vi "Give old config to New config.vi"() -> ()   [LabVIEW 2022 SP3]
uses:
  Controls/SeCrTs-Config.ctl
panel:
  in  "Config 2":T1={"AO config"=[], "AI config"=[], "DI config"=[], "DO config"=[], "TC config"=[{"Channel_Name"="", "Channel_Number"="", "Pre_Scale_min"=0.0, "Pre_Scale_max"=0.0, "units"=4, " type"=7}], "ACC config"=[], "SG config"=[], "Strain Gauge Settings"={"poisson ratio"=0.3, "nominal gage resistance"=120.0, "gage factor"=2.08}, "Bridge Settings"={"voltage excitation value"=3.3, "voltage excitation source"=10200, "initial bridge voltage"=0.0, "lead wire resistance"=1.7, "strain configuration"=10271}, "Sample Rate"={"AI Sample Rate"=[], "AO Sample Rate"=[], "DI Sample Rate"=[], "TC Sample Rate"=[], "DO Sample Rate"=[], "SG Sample Rate"=[], "ACC Sample Rate"=[]}} {"Bridge Settings"."strain configuration" items=["Full Bridge I"=10183, "Full Bridge II"=10184, "Full Bridge III"=10185, "Half Bridge I"=10188, "Half Bridge II"=10189, "Quarter Bridge I"=10271, "Quarter Bridge II"=10272]; "Bridge Settings"."voltage excitation source" items=["Internal"=10200, "External"=10167, "None"=10230]; "ACC config"."Terminal configuration" items=["default"=-1, "RSE"=10083, "NRSE"=10078, "Differential"=10106, "Pseudodifferential"=12529]; "ACC config"."Sensitivity units" items=["mVolts/g"=12509, "Volts/g"=12510]; "TC config"."type" items=["J"=10072, "K"=10073, "N"=10077, "R"=10082, "S"=10085, "T"=10086, "B"=10047, "E"=10055]; "TC config"."units" items=["Deg C", "Deg F", "Kelvins", "Deg R", "From Custom Scale"]}
  out "output cluster":T1={"AO config"=[], "AI config"=[], "DI config"=[], "DO config"=[], "TC config"=[], "ACC config"=[], "SG config"=[], "Strain Gauge Settings"={"poisson ratio"=0.3, "nominal gage resistance"=120.0, "gage factor"=2.08}, "Bridge Settings"={"voltage excitation value"=3.3, "voltage excitation source"=10200, "initial bridge voltage"=0.0, "lead wire resistance"=1.7, "strain configuration"=10271}, "Sample Rate"={"AI Sample Rate"=[], "AO Sample Rate"=[], "DI Sample Rate"=[], "TC Sample Rate"=[], "DO Sample Rate"=[], "SG Sample Rate"=[], "ACC Sample Rate"=[]}} {"Bridge Settings"."strain configuration" items=["Full Bridge I"=10183, "Full Bridge II"=10184, "Full Bridge III"=10185, "Half Bridge I"=10188, "Half Bridge II"=10189, "Quarter Bridge I"=10271, "Quarter Bridge II"=10272]; "Bridge Settings"."voltage excitation source" items=["Internal"=10200, "External"=10167, "None"=10230]; "ACC config"."Terminal configuration" items=["default"=-1, "RSE"=10083, "NRSE"=10078, "Differential"=10106, "Pseudodifferential"=12529]; "ACC config"."Sensitivity units" items=["mVolts/g"=12509, "Volts/g"=12510]; "TC config"."type" items=["J"=10072, "K"=10073, "N"=10077, "R"=10082, "S"=10085, "T"=10086, "B"=10047, "E"=10055]; "TC config"."units" items=["Deg C", "Deg F", "Kelvins", "Deg R", "From Custom Scale"]}
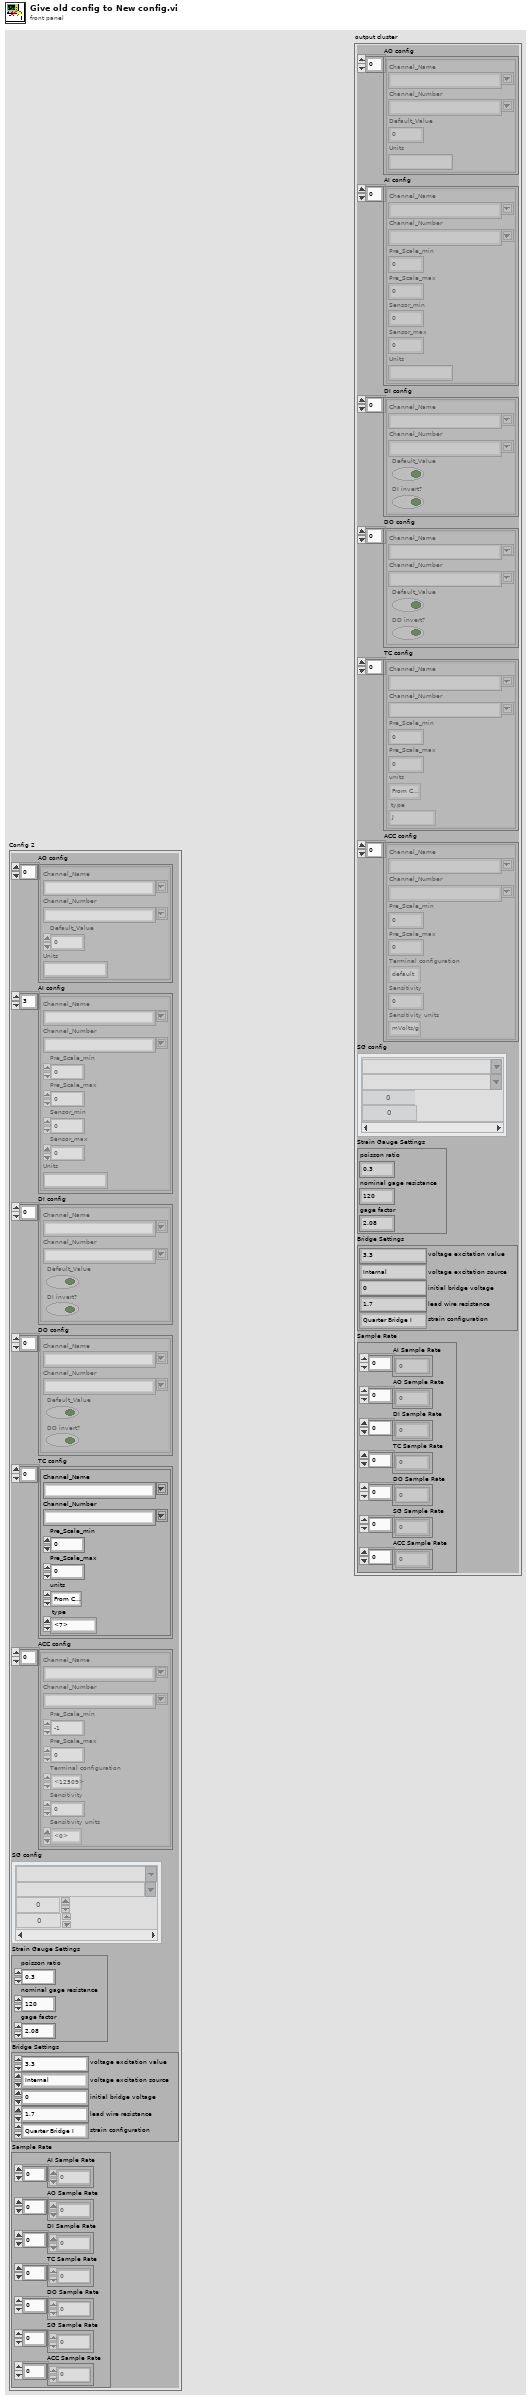
[diagram p1: front panel]
types:
  T1 = typedef "SeCrTs-Config.ctl" = cluster{"AO config":cluster{"Channel_Name":string, "Channel_Number":string, "Default_Value":dbl, "Units":string}[], "AI config":cluster{"Channel_Name":string, "Channel_Number":string, "Pre_Scale_min":dbl, "Pre_Scale_max":dbl, "Sensor_min":dbl, "Sensor_max":dbl, "Units":string}[], "DI config":cluster{"Channel_Name":string, "Channel_Number":string, "Default_Value":bool, "DI invert?":bool}[], "DO config":cluster{"Channel_Name":string, "Channel_Number":string, "Default_Value":bool, "DO invert?":bool}[], "TC config":cluster{"Channel_Name":string, "Channel_Number":string, "Pre_Scale_min":dbl, "Pre_Scale_max":dbl, "units":i32, " type":i32}[], "ACC config":cluster{"Channel_Name":string, "Channel_Number":string, "Pre_Scale_min":dbl, "Pre_Scale_max":dbl, "Terminal configuration":i32, "Sensitivity":dbl, "Sensitivity units":i32}[], "SG config":cluster{"Channel_Name":string, "Channel_Number":string, "Pre_Scale_min":dbl, "Pre_Scale_max":dbl}[], "Strain Gauge Settings":cluster{"poisson ratio":dbl, "nominal gage resistance":dbl, "gage factor":dbl}, "Bridge Settings":cluster{"voltage excitation value":dbl, "voltage excitation source":i32, "initial bridge voltage":dbl, "lead wire resistance":dbl, "strain configuration":i32}, "Sample Rate":cluster{"AI Sample Rate":dbl[], "AO Sample Rate":dbl[], "DI Sample Rate":dbl[], "TC Sample Rate":dbl[], "DO Sample Rate":dbl[], "SG Sample Rate":dbl[], "ACC Sample Rate":dbl[]}}
  T2 = cluster{cluster{"AI":cluster{"AI signal Lists":string, "AI Channel List":string, "Prescale Min":dbl, "Prescale Max":dbl, "Prescale Unit":string, "Sensor Min":dbl, "Sensor Max":dbl, "Sensor Unit":string}[], "AI Sample rate":u32[], "AI Device list ":string[]}, cluster{"AO":cluster{"AO signal List":string, "AO Channel List":string, "AO Default Value":dbl}[], "AO Sample rate ":u32[], "AO Device list":string[]}, cluster{"DI":cluster{"DI Signal List":string, "DI Channel list":string, "Default":bool, "Inverted":bool}[], "DI Sample rate":u32[], "DI Device list  ":string[]}, cluster{"DO":cluster{"DO Signal List":string, "DO Channel List":string, "DO Default":bool, "DO Inverted":bool}[], "DO Sample rate":u32[], "DO Device list ":string[]}, cluster{"CI":cluster{"CI Signal list":string, "CI Channel List":string, "Initial Count":u32, "Count Direction":i32, "Edge":i32}[], "CI Sample rate":u32[], "CI Device list ":string[]}, cluster{"TC":cluster{"TC signal Lists":string, "TC Channel Lists":string, "TC type":i32, "Max.Value":dbl, "Min.Value":dbl, "Units":i32}[], "TC Sample rate":u32[], "TC Device list":string[]}, cluster{"Accelerometer":cluster{"name to assign":string, "physical channels":tag, "minimum value":dbl, "maximum value":dbl, "sensitivity":dbl, "sensitivity units":i32, "units":i32}[], "Acc Sampling Rate":string}}
  T3 = cluster{"AI":cluster{"AI signal Lists":string, "AI Channel List":string, "Prescale Min":dbl, "Prescale Max":dbl, "Prescale Unit":string, "Sensor Min":dbl, "Sensor Max":dbl, "Sensor Unit":string}[], "AI Sample rate":u32[], "AI Device list ":string[]}
  T4 = cluster{"AO":cluster{"AO signal List":string, "AO Channel List":string, "AO Default Value":dbl}[], "AO Sample rate ":u32[], "AO Device list":string[]}
  T5 = cluster{"DI":cluster{"DI Signal List":string, "DI Channel list":string, "Default":bool, "Inverted":bool}[], "DI Sample rate":u32[], "DI Device list  ":string[]}
  T6 = cluster{"DO":cluster{"DO Signal List":string, "DO Channel List":string, "DO Default":bool, "DO Inverted":bool}[], "DO Sample rate":u32[], "DO Device list ":string[]}
  T7 = cluster{"TC":cluster{"TC signal Lists":string, "TC Channel Lists":string, "TC type":i32, "Max.Value":dbl, "Min.Value":dbl, "Units":i32}[], "TC Sample rate":u32[], "TC Device list":string[]}
  T8 = cluster{"Accelerometer":cluster{"name to assign":string, "physical channels":tag, "minimum value":dbl, "maximum value":dbl, "sensitivity":dbl, "sensitivity units":i32, "units":i32}[], "Acc Sampling Rate":string}
  T9 = cluster{"name to assign":string, "physical channels":tag, "minimum value":dbl, "maximum value":dbl, "sensitivity":dbl, "sensitivity units":i32, "units":i32}[]
  T10 = cluster{"AO signal List":string, "AO Channel List":string, "AO Default Value":dbl}[]
  T11 = cluster{"DO Signal List":string, "DO Channel List":string, "DO Default":bool, "DO Inverted":bool}[]
  T12 = cluster{"TC signal Lists":string, "TC Channel Lists":string, "TC type":i32, "Max.Value":dbl, "Min.Value":dbl, "Units":i32}[]
  T13 = cluster{"AI signal Lists":string, "AI Channel List":string, "Prescale Min":dbl, "Prescale Max":dbl, "Prescale Unit":string, "Sensor Min":dbl, "Sensor Max":dbl, "Sensor Unit":string}[]
  T14 = cluster{"DI Signal List":string, "DI Channel list":string, "Default":bool, "Inverted":bool}[]
  T15 = cluster{"Channel_Name":string, "Channel_Number":string, "Pre_Scale_min":dbl, "Pre_Scale_max":dbl, "units":i32, " type":i32}
  T16 = cluster{"Channel_Name":string, "Channel_Number":string, "Pre_Scale_min":dbl, "Pre_Scale_max":dbl, "Sensor_min":dbl, "Sensor_max":dbl, "Units":string}
  T17 = cluster{"Channel_Name":string, "Channel_Number":string, "Default_Value":dbl, "Units":string}
  T18 = cluster{"Channel_Name":string, "Channel_Number":string, "Default_Value":bool, "DI invert?":bool}
  T19 = cluster{"Channel_Name":string, "Channel_Number":string, "Pre_Scale_min":dbl, "Pre_Scale_max":dbl, "Terminal configuration":i32, "Sensitivity":dbl, "Sensitivity units":i32}
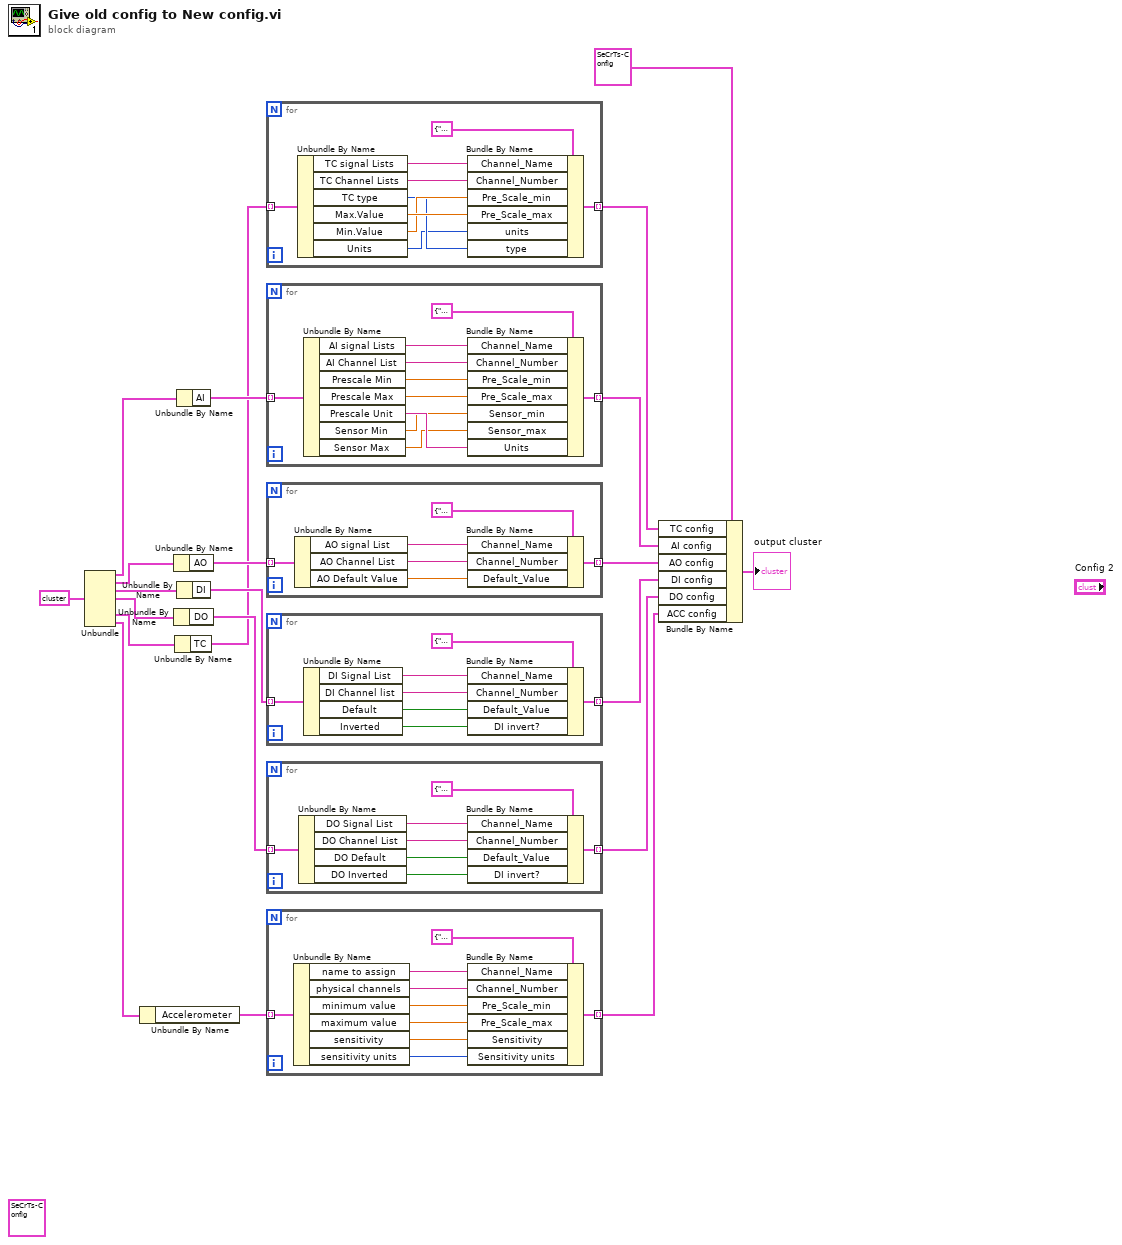
[diagram p0: block diagram]
diagram:
  (unwired) T1 {"AO config"=[{"Channel_Name"="TCV_1018", "Channel_Number"="PXI1Slot6/ao0", "Default_Value"=0.0, "Units"="Volt"}], "AI config"=[{"Channel_Name"="F_PT_1019", "Channel_Number"="PXI1Slot10/ai1", "Pre_Scale_min"=0.004, "Pre_Scale_max"=0.02, "Sensor_min"=0.0, "Sensor_max"=40.0, "Units"="bar"}, {"Channel_Name"="F_RTD_1013", "Channel_Number"="PXI1Slot10/ai2", "Pre_Scale_min"=0.004, "Pre_Scale_max"=0.02, "Sensor_min"=73.15, "Sensor_max"=373.15, "Units"="K"}, {"Channel_Name"="F_PT_1013a", "Channel_Number"="PXI1Slot10/ai3", "Pre_Scale_min"=0.004, "Pre_Scale_max"=0.02, "Sensor_min"=0.0, "Sensor_max"=200.0, "Units"="bar"}, {"Channel_Name"="F_PT_1013b", "Channel_Number"="PXI1Slot10/ai4", "Pre_Scale_min"=0.004, "Pre_Scale_max"=0.02, "Sensor_min"=0.0, "Sensor_max"=200.0, "Units"="bar"}, {"Channel_Name"="F_PT_1011a", "Channel_Number"="PXI1Slot10/ai5", "Pre_Scale_min"=0.004, "Pre_Scale_max"=0.02, "Sensor_min"=0.0, "Sensor_max"=40.0, "Units"="bar"}, {"Channel_Name"="F_PT_1011b", "Channel_Number"="PXI1Slot10/ai6", "Pre_Scale_min"=0.004, "Pre_Scale_max"=0.02, "Sensor_min"=0.0, "Sensor_max"=40.0, "Units"="bar"}, {"Channel_Name"="F_SC_RTD", "Channel_Number"="PXI1Slot10/ai7", "Pre_Scale_min"=0.004, "Pre_Scale_max"=0.02, "Sensor_min"=73.15, "Sensor_max"=373.15, "Units"="K"}, {"Channel_Name"="W_RTD_1177", "Channel_Number"="PXI1Slot10/ai8", "Pre_Scale_min"=0.004, "Pre_Scale_max"=0.02, "Sensor_min"=73.15, "Sensor_max"=773.15, "Units"="K"}, {"Channel_Name"="N_PT_1090", "Channel_Number"="PXI1Slot10/ai10", "Pre_Scale_min"=0.004, "Pre_Scale_max"=0.02, "Sensor_min"=0.0, "Sensor_max"=40.0, "Units"="bar"}, {"Channel_Name"="TCV_1018(FB)", "Channel_Number"="PXI1Slot10/ai11", "Pre_Scale_min"=0.004, "Pre_Scale_max"=0.02, "Sensor_min"=0.0, "Sensor_max"=100.0, "Units"="Percentage"}, {"Channel_Name"="F_FM-1010", "Channel_Number"="PXI1Slot10/ai12", "Pre_Scale_min"=0.004, "Pre_Scale_max"=0.02, "Sensor_min"=0.0, "Sensor_max"=10.0, "Units"="kg/s"}, {"Channel_Name"="F_PT_SC", "Channel_Number"="PXI1Slot10/ai13", "Pre_Scale_min"=0.004, "Pre_Scale_max"=0.02, "Sensor_min"=0.0, "Sensor_max"=40.0, "Units"="bar"}, {"Channel_Name"="PT 1000 - 2", "Channel_Number"="PXI1Slot10/ai14", "Pre_Scale_min"=0.004, "Pre_Scale_max"=0.02, "Sensor_min"=253.15, "Sensor_max"=453.15, "Units"="K"}, {"Channel_Name"="PT 1000 ", "Channel_Number"="PXI1Slot10/ai17", "Pre_Scale_min"=0.004, "Pre_Scale_max"=0.02, "Sensor_min"=253.15, "Sensor_max"=453.15, "Units"="K"}, {"Channel_Name"="N_PT_1101", "Channel_Number"="cRIOMod3/ai0", "Pre_Scale_min"=0.0, "Pre_Scale_max"=10.0, "Sensor_min"=0.0, "Sensor_max"=40.0, "Units"="bar"}, {"Channel_Name"="N_PT_1210", "Channel_Number"="cRIOMod3/ai1", "Pre_Scale_min"=0.0, "Pre_Scale_max"=10.0, "Sensor_min"=0.0, "Sensor_max"=100.0, "Units"="bar"}, {"Channel_Name"="W_PT_1212", "Channel_Number"="cRIOMod3/ai2", "Pre_Scale_min"=0.0, "Pre_Scale_max"=10.0, "Sensor_min"=0.0, "Sensor_max"=100.0, "Units"="bar"}, {"Channel_Name"="F_RTD_1212", "Channel_Number"="cRIOMod3/ai3", "Pre_Scale_min"=0.0, "Pre_Scale_max"=10.0, "Sensor_min"=73.15, "Sensor_max"=373.15, "Units"="K"}, {"Channel_Name"="Tank6", "Channel_Number"="cRIOMod3/ai4", "Pre_Scale_min"=0.0, "Pre_Scale_max"=10.0, "Sensor_min"=0.0, "Sensor_max"=290.0, "Units"="mbar"}, {"Channel_Name"="Vdc", "Channel_Number"="PXI1Slot8/ai0", "Pre_Scale_min"=-5.0, "Pre_Scale_max"=5.0, "Sensor_min"=-700.0, "Sensor_max"=700.0, "Units"="Volts"}, {"Channel_Name"="Vrms1", "Channel_Number"="PXI1Slot8/ai1", "Pre_Scale_min"=-5.0, "Pre_Scale_max"=5.0, "Sensor_min"=-700.0, "Sensor_max"=700.0, "Units"="Volts"}, {"Channel_Name"="Vrms2", "Channel_Number"="PXI1Slot8/ai2", "Pre_Scale_min"=-5.0, "Pre_Scale_max"=5.0, "Sensor_min"=-700.0, "Sensor_max"=700.0, "Units"="Volts"}, {"Channel_Name"="Vrms3", "Channel_Number"="PXI1Slot8/ai3", "Pre_Scale_min"=-5.0, "Pre_Scale_max"=5.0, "Sensor_min"=-700.0, "Sensor_max"=700.0, "Units"="Volts"}, {"Channel_Name"="Idc", "Channel_Number"="PXI1Slot8/ai4", "Pre_Scale_min"=-8.506, "Pre_Scale_max"=8.506, "Sensor_min"=-424.26, "Sensor_max"=424.26, "Units"="Volts"}, {"Channel_Name"="Irms1", "Channel_Number"="PXI1Slot8/ai5", "Pre_Scale_min"=-8.506, "Pre_Scale_max"=8.506, "Sensor_min"=-424.26, "Sensor_max"=424.26, "Units"="Volts"}, {"Channel_Name"="Irms2", "Channel_Number"="PXI1Slot8/ai6", "Pre_Scale_min"=-8.506, "Pre_Scale_max"=8.506, "Sensor_min"=-424.26, "Sensor_max"=424.26, "Units"="Volts"}, {"Channel_Name"="Irms3", "Channel_Number"="PXI1Slot8/ai7", "Pre_Scale_min"=-8.506, "Pre_Scale_max"=8.506, "Sensor_min"=-424.26, "Sensor_max"=424.26, "Units"="Volts"}, {"Channel_Name"="PT_1", "Channel_Number"="PXI1Slot10/ai19", "Pre_Scale_min"=0.004, "Pre_Scale_max"=0.02, "Sensor_min"=0.0, "Sensor_max"=200.0, "Units"="bar"}, {"Channel_Name"="PT_2", "Channel_Number"="PXI1Slot10/ai20", "Pre_Scale_min"=0.004, "Pre_Scale_max"=0.02, "Sensor_min"=0.0, "Sensor_max"=40.0, "Units"="bar"}, {"Channel_Name"="PT_3", "Channel_Number"="PXI1Slot10/ai21", "Pre_Scale_min"=0.004, "Pre_Scale_max"=0.02, "Sensor_min"=0.0, "Sensor_max"=200.0, "Units"="bar"}, {"Channel_Name"="PT_4", "Channel_Number"="PXI1Slot10/ai22", "Pre_Scale_min"=0.004, "Pre_Scale_max"=0.02, "Sensor_min"=0.0, "Sensor_max"=40.0, "Units"="bar"}, {"Channel_Name"="PT_5", "Channel_Number"="PXI1Slot10/ai23", "Pre_Scale_min"=0.004, "Pre_Scale_max"=0.02, "Sensor_min"=0.0, "Sensor_max"=200.0, "Units"="bar"}, {"Channel_Name"="PT_6", "Channel_Number"="PXI1Slot10/ai24", "Pre_Scale_min"=0.004, "Pre_Scale_max"=0.02, "Sensor_min"=0.0, "Sensor_max"=200.0, "Units"="bar"}], "DI config"=[{"Channel_Name"="NC EPV 1004 HSS", "Channel_Number"="PXI1Slot13/port0/line0", "Default_Value"=FALSE, "DI invert?"=FALSE}, {"Channel_Name"="NC EPV 1008 HSS", "Channel_Number"="PXI1Slot13/port0/line1", "Default_Value"=FALSE, "DI invert?"=FALSE}, {"Channel_Name"="NO EPV 1091 HSS", "Channel_Number"="PXI1Slot13/port0/line3", "Default_Value"=TRUE, "DI invert?"=TRUE}, {"Channel_Name"="NC EPV 1217 HSS", "Channel_Number"="PXI1Slot13/port0/line2", "Default_Value"=FALSE, "DI invert?"=FALSE}, {"Channel_Name"="NO EPV 1102 HSS", "Channel_Number"="cRIOMod2/port0/line0", "Default_Value"=TRUE, "DI invert?"=TRUE}, {"Channel_Name"="NC EPV 1211 HSS", "Channel_Number"="cRIOMod2/port0/line1", "Default_Value"=FALSE, "DI invert?"=FALSE}, {"Channel_Name"="NC EPV 1214 HSS", "Channel_Number"="cRIOMod2/port0/line2", "Default_Value"=FALSE, "DI invert?"=FALSE}, {"Channel_Name"="NO EPV 1207 HSS", "Channel_Number"="cRIOMod2/port0/line3", "Default_Value"=TRUE, "DI invert?"=TRUE}, {"Channel_Name"="ATF Incomer1", "Channel_Number"="cRIOMod2/port0/line13", "Default_Value"=FALSE, "DI invert?"=FALSE}, {"Channel_Name"="ATF Incomer2", "Channel_Number"="cRIOMod2/port0/line14", "Default_Value"=FALSE, "DI invert?"=FALSE}, {"Channel_Name"="ATF Incomer3", "Channel_Number"="cRIOMod2/port0/line20", "Default_Value"=FALSE, "DI invert?"=FALSE}, {"Channel_Name"="ATF Incomer4", "Channel_Number"="cRIOMod2/port0/line17", "Default_Value"=FALSE, "DI invert?"=FALSE}, {"Channel_Name"="ATF Incomer4R", "Channel_Number"="cRIOMod2/port0/line18", "Default_Value"=FALSE, "DI invert?"=FALSE}, {"Channel_Name"="Engine Incomer1", "Channel_Number"="cRIOMod2/port0/line15", "Default_Value"=FALSE, "DI invert?"=FALSE}, {"Channel_Name"="Engine Incomer2", "Channel_Number"="cRIOMod2/port0/line21", "Default_Value"=FALSE, "DI invert?"=FALSE}, {"Channel_Name"="Engine Incomer4", "Channel_Number"="cRIOMod2/port0/line19", "Default_Value"=FALSE, "DI invert?"=FALSE}, {"Channel_Name"="EPV Contactor", "Channel_Number"="cRIOMod2/port0/line16", "Default_Value"=FALSE, "DI invert?"=FALSE}], "DO config"=[{"Channel_Name"="NC EPV 1004", "Channel_Number"="PXI1Slot13/port2/line0", "Default_Value"=FALSE, "DO invert?"=FALSE}, {"Channel_Name"="NC EPV 1008", "Channel_Number"="PXI1Slot13/port2/line1", "Default_Value"=FALSE, "DO invert?"=FALSE}, {"Channel_Name"="NO EPV 1091", "Channel_Number"="PXI1Slot13/port2/line3", "Default_Value"=TRUE, "DO invert?"=TRUE}, {"Channel_Name"="NC EPV 1217", "Channel_Number"="PXI1Slot13/port2/line2", "Default_Value"=FALSE, "DO invert?"=FALSE}, {"Channel_Name"="NC EPV 1211", "Channel_Number"="cRIOMod1/port0/line1", "Default_Value"=FALSE, "DO invert?"=FALSE}, {"Channel_Name"="NO EPV 1102", "Channel_Number"="cRIOMod1/port0/line0", "Default_Value"=TRUE, "DO invert?"=TRUE}, {"Channel_Name"="NC EPV 1214", "Channel_Number"="cRIOMod1/port0/line2", "Default_Value"=FALSE, "DO invert?"=FALSE}, {"Channel_Name"="NO EPV 1207", "Channel_Number"="cRIOMod1/port0/line3", "Default_Value"=TRUE, "DO invert?"=TRUE}, {"Channel_Name"="Gate driver power", "Channel_Number"="PXI1Slot13/port2/line4", "Default_Value"=FALSE, "DO invert?"=FALSE}, {"Channel_Name"="MCU reset", "Channel_Number"="PXI1Slot13/port2/line5", "Default_Value"=FALSE, "DO invert?"=FALSE}, {"Channel_Name"="ADS reset", "Channel_Number"="PXI1Slot13/port2/line6", "Default_Value"=FALSE, "DO invert?"=FALSE}, {"Channel_Name"="AC Button", "Channel_Number"="cRIOMod1/port0/line15", "Default_Value"=FALSE, "DO invert?"=FALSE}], "TC config"=[{"Channel_Name"="TC1", "Channel_Number"="PXI1Slot17/ai11", "Pre_Scale_min"=0.0, "Pre_Scale_max"=200.0, "units"=10143, " type"=10073}, {"Channel_Name"="TC2", "Channel_Number"="PXI1Slot17/ai12", "Pre_Scale_min"=0.0, "Pre_Scale_max"=200.0, "units"=10143, " type"=10073}, {"Channel_Name"="TC3", "Channel_Number"="PXI1Slot17/ai13", "Pre_Scale_min"=0.0, "Pre_Scale_max"=200.0, "units"=10143, " type"=10073}, {"Channel_Name"="TC4", "Channel_Number"="PXI1Slot17/ai6", "Pre_Scale_min"=0.0, "Pre_Scale_max"=200.0, "units"=10143, " type"=10073}, {"Channel_Name"="TC5", "Channel_Number"="PXI1Slot17/ai7", "Pre_Scale_min"=0.0, "Pre_Scale_max"=200.0, "units"=10143, " type"=10073}, {"Channel_Name"="TC6", "Channel_Number"="PXI1Slot17/ai8", "Pre_Scale_min"=0.0, "Pre_Scale_max"=200.0, "units"=10143, " type"=10073}, {"Channel_Name"="TC7", "Channel_Number"="PXI1Slot17/ai9", "Pre_Scale_min"=0.0, "Pre_Scale_max"=200.0, "units"=10143, " type"=10073}, {"Channel_Name"="TC8", "Channel_Number"="PXI1Slot17/ai10", "Pre_Scale_min"=0.0, "Pre_Scale_max"=200.0, "units"=10143, " type"=10073}, {"Channel_Name"="NDEBT", "Channel_Number"="PXI1Slot17/ai0", "Pre_Scale_min"=0.0, "Pre_Scale_max"=200.0, "units"=10143, " type"=10073}, {"Channel_Name"="Motor Outer", "Channel_Number"="PXI1Slot17/ai1", "Pre_Scale_min"=0.0, "Pre_Scale_max"=200.0, "units"=10143, " type"=10073}, {"Channel_Name"="DEBT", "Channel_Number"="PXI1Slot17/ai2", "Pre_Scale_min"=0.0, "Pre_Scale_max"=200.0, "units"=10143, " type"=10073}], "ACC config"=[{"Channel_Name"="DH", "Channel_Number"="PXI1Slot12/ai0", "Pre_Scale_min"=-50.0, "Pre_Scale_max"=50.0, "Terminal configuration"=-1, "Sensitivity"=100.0, "Sensitivity units"=12509}, {"Channel_Name"="NDV", "Channel_Number"="PXI1Slot12/ai1", "Pre_Scale_min"=-50.0, "Pre_Scale_max"=50.0, "Terminal configuration"=-1, "Sensitivity"=100.0, "Sensitivity units"=12509}, {"Channel_Name"="NDH", "Channel_Number"="PXI1Slot12/ai2", "Pre_Scale_min"=-50.0, "Pre_Scale_max"=50.0, "Terminal configuration"=-1, "Sensitivity"=100.0, "Sensitivity units"=12509}, {"Channel_Name"="DV", "Channel_Number"="PXI1Slot12/ai3", "Pre_Scale_min"=-50.0, "Pre_Scale_max"=50.0, "Terminal configuration"=-1, "Sensitivity"=100.0, "Sensitivity units"=12509}, {"Channel_Name"="NDA", "Channel_Number"="PXI1Slot12/ai4", "Pre_Scale_min"=-50.0, "Pre_Scale_max"=50.0, "Terminal configuration"=-1, "Sensitivity"=100.0, "Sensitivity units"=12509}, {"Channel_Name"="DA", "Channel_Number"="PXI1Slot12/ai5", "Pre_Scale_min"=-50.0, "Pre_Scale_max"=50.0, "Terminal configuration"=-1, "Sensitivity"=100.0, "Sensitivity units"=12509}], "SG config"=[], "Strain Gauge Settings"={"poisson ratio"=0.3, "nominal gage resistance"=120.0, "gage factor"=2.08}, "Bridge Settings"={"voltage excitation value"=3.3, "voltage excitation source"=10200, "initial bridge voltage"=0.0, "lead wire resistance"=1.7, "strain configuration"=10271}, "Sample Rate"={"AI Sample Rate"=[], "AO Sample Rate"=[], "DI Sample Rate"=[], "TC Sample Rate"=[], "DO Sample Rate"=[], "SG Sample Rate"=[], "ACC Sample Rate"=[]}} ("Config 2")
  n1 = Unbundle(T2 {{"AI"=[{"AI signal Lists"="F_PT_1019", "AI Channel List"="PXI1Slot10/ai1", "Prescale Min"=0.004, "Prescale Max"=0.02, "Prescale Unit"="Amps", "Sensor Min"=0.0, "Sensor Max"=40.0, "Sensor Unit"="bar"}, {"AI signal Lists"="F_RTD_1013", "AI Channel List"="PXI1Slot10/ai2", "Prescale Min"=0.004, "Prescale Max"=0.02, "Prescale Unit"="Amps", "Sensor Min"=73.15, "Sensor Max"=373.15, "Sensor Unit"="K"}, {"AI signal Lists"="F_PT_1013a", "AI Channel List"="PXI1Slot10/ai3", "Prescale Min"=0.004, "Prescale Max"=0.02, "Prescale Unit"="Amps", "Sensor Min"=0.0, "Sensor Max"=200.0, "Sensor Unit"="bar"}, {"AI signal Lists"="F_PT_1013b", "AI Channel List"="PXI1Slot10/ai4", "Prescale Min"=0.004, "Prescale Max"=0.02, "Prescale Unit"="Amps", "Sensor Min"=0.0, "Sensor Max"=200.0, "Sensor Unit"="bar"}, {"AI signal Lists"="F_PT_1011a", "AI Channel List"="PXI1Slot10/ai5", "Prescale Min"=0.004, "Prescale Max"=0.02, "Prescale Unit"="Amps", "Sensor Min"=0.0, "Sensor Max"=40.0, "Sensor Unit"="bar"}, {"AI signal Lists"="F_PT_1011b", "AI Channel List"="PXI1Slot10/ai6", "Prescale Min"=0.004, "Prescale Max"=0.02, "Prescale Unit"="Amps", "Sensor Min"=0.0, "Sensor Max"=40.0, "Sensor Unit"="bar"}, {"AI signal Lists"="F_SC_RTD", "AI Channel List"="PXI1Slot10/ai7", "Prescale Min"=0.004, "Prescale Max"=0.02, "Prescale Unit"="Amps", "Sensor Min"=73.15, "Sensor Max"=373.15, "Sensor Unit"="K"}, {"AI signal Lists"="W_RTD_1177", "AI Channel List"="PXI1Slot10/ai8", "Prescale Min"=0.004, "Prescale Max"=0.02, "Prescale Unit"="Amps", "Sensor Min"=73.15, "Sensor Max"=773.15, "Sensor Unit"="K"}, {"AI signal Lists"="N_PT_1090", "AI Channel List"="PXI1Slot10/ai10", "Prescale Min"=0.004, "Prescale Max"=0.02, "Prescale Unit"="Amps", "Sensor Min"=0.0, "Sensor Max"=40.0, "Sensor Unit"="bar"}, {"AI signal Lists"="TCV_1018(FB)", "AI Channel List"="PXI1Slot10/ai11", "Prescale Min"=0.004, "Prescale Max"=0.02, "Prescale Unit"="Amps", "Sensor Min"=0.0, "Sensor Max"=100.0, "Sensor Unit"="percentage"}, {"AI signal Lists"="F_FM-1010", "AI Channel List"="PXI1Slot10/ai12", "Prescale Min"=0.004, "Prescale Max"=0.02, "Prescale Unit"="Amps", "Sensor Min"=0.0, "Sensor Max"=10.0, "Sensor Unit"="kg/s"}, {"AI signal Lists"="F_PT_SC", "AI Channel List"="PXI1Slot10/ai13", "Prescale Min"=0.004, "Prescale Max"=0.02, "Prescale Unit"="Amps", "Sensor Min"=0.0, "Sensor Max"=40.0, "Sensor Unit"="bar"}, {"AI signal Lists"="PT 1000 - 2", "AI Channel List"="PXI1Slot10/ai14", "Prescale Min"=0.004, "Prescale Max"=0.02, "Prescale Unit"="Amps", "Sensor Min"=253.15, "Sensor Max"=453.15, "Sensor Unit"="Kelvin"}, {"AI signal Lists"="PT 1000 ", "AI Channel List"="PXI1Slot10/ai17", "Prescale Min"=0.004, "Prescale Max"=0.02, "Prescale Unit"="Amps", "Sensor Min"=253.15, "Sensor Max"=453.15, "Sensor Unit"="Kelvin"}, {"AI signal Lists"="N_PT_1101", "AI Channel List"="cRIOMod3/ai0", "Prescale Min"=0.0, "Prescale Max"=10.0, "Prescale Unit"="Volts", "Sensor Min"=0.0, "Sensor Max"=40.0, "Sensor Unit"="bar"}, {"AI signal Lists"="N_PT_1210", "AI Channel List"="cRIOMod3/ai1", "Prescale Min"=0.0, "Prescale Max"=10.0, "Prescale Unit"="Volts", "Sensor Min"=0.0, "Sensor Max"=100.0, "Sensor Unit"="bar"}, {"AI signal Lists"="W_PT_1212", "AI Channel List"="cRIOMod3/ai2", "Prescale Min"=0.0, "Prescale Max"=10.0, "Prescale Unit"="Volts", "Sensor Min"=0.0, "Sensor Max"=100.0, "Sensor Unit"="bar"}, {"AI signal Lists"="F_RTD_1212", "AI Channel List"="cRIOMod3/ai3", "Prescale Min"=0.0, "Prescale Max"=10.0, "Prescale Unit"="Volts", "Sensor Min"=73.15, "Sensor Max"=373.15, "Sensor Unit"="K"}, {"AI signal Lists"="Tank6", "AI Channel List"="cRIOMod3/ai4", "Prescale Min"=0.0, "Prescale Max"=10.0, "Prescale Unit"="Volts", "Sensor Min"=0.0, "Sensor Max"=290.0, "Sensor Unit"="mbar"}, {"AI signal Lists"="Vdc", "AI Channel List"="PXI1Slot8/ai0", "Prescale Min"=-5.0, "Prescale Max"=5.0, "Prescale Unit"="Volts", "Sensor Min"=-700.0, "Sensor Max"=700.0, "Sensor Unit"="V"}, {"AI signal Lists"="Vrms1", "AI Channel List"="PXI1Slot8/ai1", "Prescale Min"=-5.0, "Prescale Max"=5.0, "Prescale Unit"="Volts", "Sensor Min"=-700.0, "Sensor Max"=700.0, "Sensor Unit"="V"}, {"AI signal Lists"="Vrms2", "AI Channel List"="PXI1Slot8/ai2", "Prescale Min"=-5.0, "Prescale Max"=5.0, "Prescale Unit"="Volts", "Sensor Min"=-700.0, "Sensor Max"=700.0, "Sensor Unit"="V"}, {"AI signal Lists"="Vrms3", "AI Channel List"="PXI1Slot8/ai3", "Prescale Min"=-5.0, "Prescale Max"=5.0, "Prescale Unit"="Volts", "Sensor Min"=-700.0, "Sensor Max"=700.0, "Sensor Unit"="V"}, {"AI signal Lists"="Idc", "AI Channel List"="PXI1Slot8/ai4", "Prescale Min"=-8.506, "Prescale Max"=8.506, "Prescale Unit"="Volts", "Sensor Min"=-424.26, "Sensor Max"=424.26, "Sensor Unit"="V"}, {"AI signal Lists"="Irms1", "AI Channel List"="PXI1Slot8/ai5", "Prescale Min"=-8.506, "Prescale Max"=8.506, "Prescale Unit"="Volts", "Sensor Min"=-424.26, "Sensor Max"=424.26, "Sensor Unit"="V"}, {"AI signal Lists"="Irms2", "AI Channel List"="PXI1Slot8/ai6", "Prescale Min"=-8.506, "Prescale Max"=8.506, "Prescale Unit"="Volts", "Sensor Min"=-424.26, "Sensor Max"=424.26, "Sensor Unit"="V"}, {"AI signal Lists"="Irms3", "AI Channel List"="PXI1Slot8/ai7", "Prescale Min"=-8.506, "Prescale Max"=8.506, "Prescale Unit"="Volts", "Sensor Min"=-424.26, "Sensor Max"=424.26, "Sensor Unit"="V"}, {"AI signal Lists"="PT_1", "AI Channel List"="PXI1Slot10/ai19", "Prescale Min"=0.004, "Prescale Max"=0.02, "Prescale Unit"="Amps", "Sensor Min"=0.0, "Sensor Max"=200.0, "Sensor Unit"="bar"}, {"AI signal Lists"="PT_2", "AI Channel List"="PXI1Slot10/ai20", "Prescale Min"=0.004, "Prescale Max"=0.02, "Prescale Unit"="Amps", "Sensor Min"=0.0, "Sensor Max"=40.0, "Sensor Unit"="bar"}, {"AI signal Lists"="PT_3", "AI Channel List"="PXI1Slot10/ai21", "Prescale Min"=0.004, "Prescale Max"=0.02, "Prescale Unit"="Amps", "Sensor Min"=0.0, "Sensor Max"=200.0, "Sensor Unit"="bar"}, {"AI signal Lists"="PT_4", "AI Channel List"="PXI1Slot10/ai22", "Prescale Min"=0.004, "Prescale Max"=0.02, "Prescale Unit"="Amps", "Sensor Min"=0.0, "Sensor Max"=40.0, "Sensor Unit"="bar"}, {"AI signal Lists"="PT_5", "AI Channel List"="PXI1Slot10/ai23", "Prescale Min"=0.004, "Prescale Max"=0.02, "Prescale Unit"="Amps", "Sensor Min"=0.0, "Sensor Max"=200.0, "Sensor Unit"="bar"}, {"AI signal Lists"="PT_6", "AI Channel List"="PXI1Slot10/ai24", "Prescale Min"=0.004, "Prescale Max"=0.02, "Prescale Unit"="Amps", "Sensor Min"=0.0, "Sensor Max"=200.0, "Sensor Unit"="bar"}], "AI Sample rate"=[1000, 1000, 1000, 1000, 1000, 1000], "AI Device list "=["ATF-Pump-Mod1", "ATF-Pump-Mod2", "ATF-Pump-Mod6", "ATF-Pump-Mod7"]}, {"AO"=[{"AO signal List"="TCV_1018", "AO Channel List"="PXI1Slot6/ao0", "AO Default Value"=0.0}], "AO Sample rate "=[1000], "AO Device list"=["ATF-Pump-Mod5"]}, {"DI"=[{"DI Signal List"="NC EPV 1004 HSS", "DI Channel list"="PXI1Slot13/port0/line0", "Default"=FALSE, "Inverted"=FALSE}, {"DI Signal List"="NC EPV 1008 HSS", "DI Channel list"="PXI1Slot13/port0/line1", "Default"=FALSE, "Inverted"=FALSE}, {"DI Signal List"="NO EPV 1091 HSS", "DI Channel list"="PXI1Slot13/port0/line3", "Default"=TRUE, "Inverted"=TRUE}, {"DI Signal List"="NC EPV 1217 HSS", "DI Channel list"="PXI1Slot13/port0/line2", "Default"=FALSE, "Inverted"=FALSE}, {"DI Signal List"="NO EPV 1102 HSS", "DI Channel list"="cRIOMod2/port0/line0", "Default"=TRUE, "Inverted"=TRUE}, {"DI Signal List"="NC EPV 1211 HSS", "DI Channel list"="cRIOMod2/port0/line1", "Default"=FALSE, "Inverted"=FALSE}, {"DI Signal List"="NC EPV 1214 HSS", "DI Channel list"="cRIOMod2/port0/line2", "Default"=FALSE, "Inverted"=FALSE}, {"DI Signal List"="NO EPV 1207 HSS", "DI Channel list"="cRIOMod2/port0/line3", "Default"=TRUE, "Inverted"=TRUE}, {"DI Signal List"="ATF Incomer1", "DI Channel list"="cRIOMod2/port0/line13", "Default"=FALSE, "Inverted"=FALSE}, {"DI Signal List"="ATF Incomer2", "DI Channel list"="cRIOMod2/port0/line14", "Default"=FALSE, "Inverted"=FALSE}, {"DI Signal List"="ATF Incomer3", "DI Channel list"="cRIOMod2/port0/line20", "Default"=FALSE, "Inverted"=FALSE}, {"DI Signal List"="ATF Incomer4", "DI Channel list"="cRIOMod2/port0/line17", "Default"=FALSE, "Inverted"=FALSE}, {"DI Signal List"="ATF Incomer4R", "DI Channel list"="cRIOMod2/port0/line18", "Default"=FALSE, "Inverted"=FALSE}, {"DI Signal List"="Engine Incomer1", "DI Channel list"="cRIOMod2/port0/line15", "Default"=FALSE, "Inverted"=FALSE}, {"DI Signal List"="Engine Incomer2", "DI Channel list"="cRIOMod2/port0/line21", "Default"=FALSE, "Inverted"=FALSE}, {"DI Signal List"="Engine Incomer4", "DI Channel list"="cRIOMod2/port0/line19", "Default"=FALSE, "Inverted"=FALSE}, {"DI Signal List"="EPV Contactor", "DI Channel list"="cRIOMod2/port0/line16", "Default"=FALSE, "Inverted"=FALSE}], "DI Sample rate"=[1000, 1000, 1000, 1000, 1000], "DI Device list  "=["ATF-Pump-Mod3", "ATF-Pump-Mod4"]}, {"DO"=[{"DO Signal List"="NC EPV 1004", "DO Channel List"="PXI1Slot13/port2/line0", "DO Default"=FALSE, "DO Inverted"=FALSE}, {"DO Signal List"="NC EPV 1008", "DO Channel List"="PXI1Slot13/port2/line1", "DO Default"=FALSE, "DO Inverted"=FALSE}, {"DO Signal List"="NO EPV 1091", "DO Channel List"="PXI1Slot13/port2/line3", "DO Default"=TRUE, "DO Inverted"=TRUE}, {"DO Signal List"="NC EPV 1217", "DO Channel List"="PXI1Slot13/port2/line2", "DO Default"=FALSE, "DO Inverted"=FALSE}, {"DO Signal List"="NC EPV 1211", "DO Channel List"="cRIOMod1/port0/line1", "DO Default"=FALSE, "DO Inverted"=FALSE}, {"DO Signal List"="NO EPV 1102", "DO Channel List"="cRIOMod1/port0/line0", "DO Default"=TRUE, "DO Inverted"=TRUE}, {"DO Signal List"="NC EPV 1214", "DO Channel List"="cRIOMod1/port0/line2", "DO Default"=FALSE, "DO Inverted"=FALSE}, {"DO Signal List"="NO EPV 1207", "DO Channel List"="cRIOMod1/port0/line3", "DO Default"=TRUE, "DO Inverted"=TRUE}, {"DO Signal List"="Gate driver power", "DO Channel List"="PXI1Slot13/port2/line4", "DO Default"=FALSE, "DO Inverted"=FALSE}, {"DO Signal List"="MCU reset", "DO Channel List"="PXI1Slot13/port2/line5", "DO Default"=FALSE, "DO Inverted"=FALSE}, {"DO Signal List"="ADS reset", "DO Channel List"="PXI1Slot13/port2/line6", "DO Default"=FALSE, "DO Inverted"=FALSE}, {"DO Signal List"="AC Button", "DO Channel List"="cRIOMod1/port0/line15", "DO Default"=FALSE, "DO Inverted"=FALSE}], "DO Sample rate"=[1000, 1000, 1000, 1000, 1000], "DO Device list "=["ATF-Pump-Mod3", "ATF-Pump-Mod4"]}, {"CI"=[], "CI Sample rate"=[1000, 1000], "CI Device list "=[]}, {"TC"=[{"TC signal Lists"="TC1", "TC Channel Lists"="PXI1Slot17/ai11", "TC type"=10073, "Max.Value"=0.0, "Min.Value"=200.0, "Units"=10143}, {"TC signal Lists"="TC2", "TC Channel Lists"="PXI1Slot17/ai12", "TC type"=10073, "Max.Value"=0.0, "Min.Value"=200.0, "Units"=10143}, {"TC signal Lists"="TC3", "TC Channel Lists"="PXI1Slot17/ai13", "TC type"=10073, "Max.Value"=0.0, "Min.Value"=200.0, "Units"=10143}, {"TC signal Lists"="TC4", "TC Channel Lists"="PXI1Slot17/ai6", "TC type"=10073, "Max.Value"=0.0, "Min.Value"=200.0, "Units"=10143}, {"TC signal Lists"="TC5", "TC Channel Lists"="PXI1Slot17/ai7", "TC type"=10073, "Max.Value"=0.0, "Min.Value"=200.0, "Units"=10143}, {"TC signal Lists"="TC6", "TC Channel Lists"="PXI1Slot17/ai8", "TC type"=10073, "Max.Value"=0.0, "Min.Value"=200.0, "Units"=10143}, {"TC signal Lists"="TC7", "TC Channel Lists"="PXI1Slot17/ai9", "TC type"=10073, "Max.Value"=0.0, "Min.Value"=200.0, "Units"=10143}, {"TC signal Lists"="TC8", "TC Channel Lists"="PXI1Slot17/ai10", "TC type"=10073, "Max.Value"=0.0, "Min.Value"=200.0, "Units"=10143}, {"TC signal Lists"="NDEBT", "TC Channel Lists"="PXI1Slot17/ai0", "TC type"=10073, "Max.Value"=0.0, "Min.Value"=200.0, "Units"=10143}, {"TC signal Lists"="Motor Outer", "TC Channel Lists"="PXI1Slot17/ai1", "TC type"=10073, "Max.Value"=0.0, "Min.Value"=200.0, "Units"=10143}, {"TC signal Lists"="DEBT", "TC Channel Lists"="PXI1Slot17/ai2", "TC type"=10073, "Max.Value"=0.0, "Min.Value"=200.0, "Units"=10143}], "TC Sample rate"=[100, 100], "TC Device list"=[]}, {"Accelerometer"=[{"name to assign"="DH", "physical channels"="PXI1Slot12/ai0", "minimum value"=-50.0, "maximum value"=50.0, "sensitivity"=100.0, "sensitivity units"=12509, "units"=10186}, {"name to assign"="NDV", "physical channels"="PXI1Slot12/ai1", "minimum value"=-50.0, "maximum value"=50.0, "sensitivity"=100.0, "sensitivity units"=12509, "units"=10186}, {"name to assign"="NDH", "physical channels"="PXI1Slot12/ai2", "minimum value"=-50.0, "maximum value"=50.0, "sensitivity"=100.0, "sensitivity units"=12509, "units"=10186}, {"name to assign"="DV", "physical channels"="PXI1Slot12/ai3", "minimum value"=-50.0, "maximum value"=50.0, "sensitivity"=100.0, "sensitivity units"=12509, "units"=10186}, {"name to assign"="NDA", "physical channels"="PXI1Slot12/ai4", "minimum value"=-50.0, "maximum value"=50.0, "sensitivity"=100.0, "sensitivity units"=12509, "units"=10186}, {"name to assign"="DA", "physical channels"="PXI1Slot12/ai5", "minimum value"=-50.0, "maximum value"=50.0, "sensitivity"=100.0, "sensitivity units"=12509, "units"=10186}], "Acc Sampling Rate"="20 kS/s"}} ("Configuration Cluster")) -> (w20:T3, w17:T4, w19:T5, w18:T6, w15:T7, w16:T8)  [unwired: 1 out]
  n2 = Unbundle By Name(w16) -> ("Accelerometer"=w5:T9)
  n3 = Unbundle By Name(w17) -> ("AO"=w11:T10)
  n4 = Unbundle By Name(w18) -> ("DO"=w7:T11)
  n5 = Unbundle By Name(w15) -> ("TC"=w3:T12)
  n6 = Unbundle By Name(w20) -> ("AI"=w12:T13)
  n7 = Unbundle By Name(w19) -> ("DI"=w9:T14)
  n8 = for {
    tunnel: [w30] -> w2 mode=indexing
    tunnel: w3 -> [w29] mode=indexing
    n9 = Unbundle By Name(w29) -> ("TC signal Lists"=w27:string, "TC Channel Lists"=w26:string, "TC type"=w23:i32, "Max.Value"=w25:dbl, "Min.Value"=w24:dbl, "Units"=w22:i32)
    n10 = Bundle By Name(cluster=T15 {"Channel_Name"="", "Channel_Number"="", "Pre_Scale_min"=0.0, "Pre_Scale_max"=0.0, "units"=0, " type"=0} ("AI"), "Channel_Name"=w27, "Channel_Number"=w26, "Pre_Scale_min"=w24, "Pre_Scale_max"=w25, "units"=w22, "type"=w23) -> (w30:T15)
  }
  n11 = for {
    tunnel: [w39] -> w13 mode=indexing
    tunnel: w12 -> [w38] mode=indexing
    n12 = Unbundle By Name(w38) -> ("AI signal Lists"=w37:string, "AI Channel List"=w36:string, "Prescale Min"=w35:dbl, "Prescale Max"=w34:dbl, "Prescale Unit"=w33:string, "Sensor Min"=w32:dbl, "Sensor Max"=w31:dbl)
    n13 = Bundle By Name(cluster=T16 {"Channel_Name"="", "Channel_Number"="", "Pre_Scale_min"=0.0, "Pre_Scale_max"=0.0, "Sensor_min"=0.0, "Sensor_max"=0.0, "Units"=""} ("AI"), "Channel_Name"=w37, "Channel_Number"=w36, "Pre_Scale_min"=w35, "Pre_Scale_max"=w34, "Sensor_min"=w32, "Sensor_max"=w31, "Units"=w33) -> (w39:T16)
  }
  n14 = for {
    tunnel: [w46] -> w10 mode=indexing
    tunnel: w11 -> [w45] mode=indexing
    n15 = Unbundle By Name(w45) -> ("AO signal List"=w44:string, "AO Channel List"=w43:string, "AO Default Value"=w42:dbl)
    n16 = Bundle By Name(cluster=T17 {"Channel_Name"="", "Channel_Number"="", "Default_Value"=0.0, "Units"=""} ("AI"), "Channel_Name"=w44, "Channel_Number"=w43, "Default_Value"=w42) -> (w46:T17)
  }
  n17 = for {
    tunnel: [w53] -> w8 mode=indexing
    tunnel: w9 -> [w52] mode=indexing
    n18 = Unbundle By Name(w52) -> ("DI Signal List"=w51:string, "DI Channel list"=w50:string, "Default"=w48:bool, "Inverted"=w47:bool)
    n19 = Bundle By Name(cluster=T18 {"Channel_Name"="", "Channel_Number"="", "Default_Value"=FALSE, "DI invert?"=FALSE} ("AI"), "Channel_Name"=w51, "Channel_Number"=w50, "Default_Value"=w48, "DI invert?"=w47) -> (w53:T18)
  }
  n20 = for {
    tunnel: [w60] -> w6 mode=indexing
    tunnel: w7 -> [w59] mode=indexing
    n21 = Unbundle By Name(w59) -> ("DO Signal List"=w58:string, "DO Channel List"=w57:string, "DO Default"=w55:bool, "DO Inverted"=w54:bool)
    n22 = Bundle By Name(cluster=T18 {"Channel_Name"="", "Channel_Number"="", "Default_Value"=FALSE, "DI invert?"=FALSE} ("AI"), "Channel_Name"=w58, "Channel_Number"=w57, "Default_Value"=w55, "DI invert?"=w54) -> (w60:T18)
  }
  n23 = for {
    tunnel: [w69] -> w4 mode=indexing
    tunnel: w5 -> [w68] mode=indexing
    n24 = Unbundle By Name(w68) -> ("name to assign"=w67:string, "physical channels"=w66:tag, "minimum value"=w64:dbl, "maximum value"=w63:dbl, "sensitivity"=w61:dbl, "sensitivity units"=w62:i32)
    n25 = Bundle By Name(cluster=T19 {"Channel_Name"="", "Channel_Number"="", "Pre_Scale_min"=0.0, "Pre_Scale_max"=0.0, "Terminal configuration"=0, "Sensitivity"=0.0, "Sensitivity units"=0} ("AI"), "Channel_Name"=w67, "Channel_Number"=w66, "Pre_Scale_min"=w64, "Pre_Scale_max"=w63, "Sensitivity"=w61, "Sensitivity units"=w62) -> (w69:T19)
  }
  n26 = Bundle By Name(cluster=T1 {"AO config"=[], "AI config"=[], "DI config"=[], "DO config"=[], "TC config"=[], "ACC config"=[], "SG config"=[], "Strain Gauge Settings"={"poisson ratio"=0.3, "nominal gage resistance"=120.0, "gage factor"=2.08}, "Bridge Settings"={"voltage excitation value"=3.3, "voltage excitation source"=10200, "initial bridge voltage"=0.0, "lead wire resistance"=1.7, "strain configuration"=10271}, "Sample Rate"={"AI Sample Rate"=[], "AO Sample Rate"=[], "DI Sample Rate"=[], "TC Sample Rate"=[], "DO Sample Rate"=[], "SG Sample Rate"=[], "ACC Sample Rate"=[]}} ("output cluster"), "TC config"=w2, "AI config"=w13, "AO config"=w10, "DI config"=w8, "DO config"=w6, "ACC config"=w4) -> (→"output cluster":T1)
